vi "Low-Level Write.vi"(5 "Finished? (True)":bool=TRUE, 6 "Mask payload?":bool, 7 "Opcode (Text)":T1=1 items=["Cont. Frame"=0, "Text"=1, "Binary"=2, "Ping"=9, "Pong"=10], 8 "error in (no error)":errorcluster, 9 "timeout ms (5000)":i32=5000, 10 "Data":u8[](array[numeric]), 11 "WebSockets in":refnum<class "WebSocket.lvclass">) -> (0 "error out":errorcluster, 1 "timed out?":bool, 3 "WebSockets out":refnum<class "WebSocket.lvclass">)   [LabVIEW 2021, in "WebSockets.lvlib" / "WebSocket.lvclass"]
doc: "Sends a WebSocket frame to the connection endpoint. Messages sent from the client must be masked but it is optional for the server.\n\nFinished should be set to True unless sending a fragmented message.\nWebSockets 2.0.1.40\nSam Sharp - MediaMongrels Ltd\nCopyright (c) 2019, MediaMongrels Ltd"
uses:
  WebSocket.lvclass
  Opcodes.ctl
  WebSocket.lvclass/WebSocket.ctl
  Sockets/Socket/Socket.lvclass
panel:
  # "(leave as 'True' unless sending fragmented messages)"
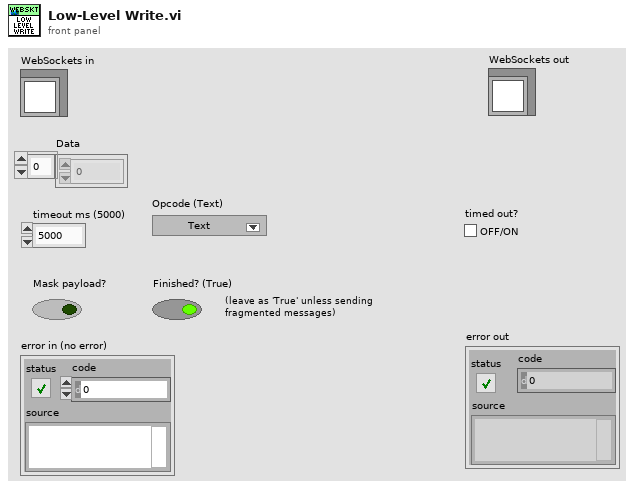
[diagram p1: front panel]
types:
  T1 = typedef "WebSockets.lvlib/WebSocket.lvclass/Opcodes.ctl" = u8
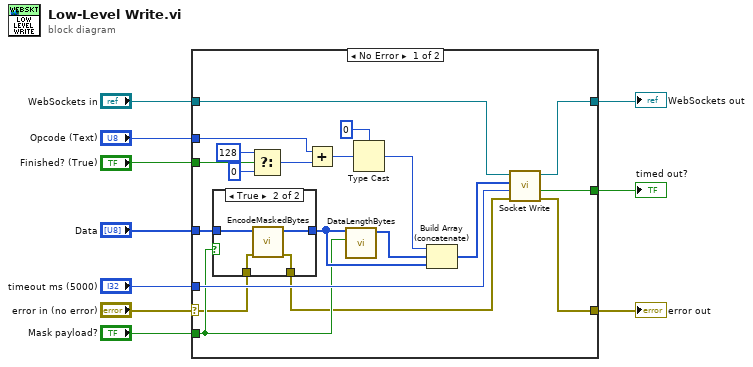
[diagram p0: block diagram]
diagram:
  n1 = case shown="No Error" "error in (no error)" {
    selector: "error in (no error)" -> [w22 w38]
    tunnel: [w30 w38] -> w9
    tunnel: [w12 w37] -> w3
    tunnel: "WebSockets in" -> [w13 w37]
    tunnel: "Data" -> [w25 _]
    tunnel: "timeout ms (5000)" -> [w26 _]
    tunnel: "Mask payload?" -> [w23 _]
    tunnel: "Finished? (True)" -> [w20 _]
    tunnel: "Opcode (Text)" -> [w18 _]
    tunnel: [w11 _] -> w1
    frame No Error {
      n2 = case shown="True" w23 {
        tunnel: w25 -> [w32 w36]
        tunnel: [w32 w35] -> w24
        tunnel: w22 -> [w31 w34]
        tunnel: [w31 w33] -> w21
        frame False {
        }
        frame True {
          n3 = call "EncodeMaskedBytes.vi"("error in (no error)"=w34, "Raw Data"=w36) -> ("error out"=w33:errorcluster, "Masked Data"=w35:u8[])  [unwired: 8 in]
        }
      }
      n4 = Select(t=u8 128, s=w20, f=u8 0) -> (s? t:f=w19:u8)
      n5 = Add(x=w18, y=w19) -> (x+y=w28:T1)
      n6 = call "DataLengthBytes.vi"("Is masked?"=w23, "Data"=w24) -> ("Length Bytes"=w29:u8[])  [unwired: 9 in]
      n7 = Type Cast(type=u8 0 ("f"), x=w28) -> (*(type *) &x=w15:u8)
      n8 = Build Array (concatenate)(w15, w29, w24) -> (w27:u8[])
      n9 = call "Socket Write.vi"("error in (no error)"=w21, "timeout ms (5000)"=w26, "Bytes to write"=w27, "WebSocket in"=w13) -> ("error out"=w30:errorcluster, "timed out?"=w11:bool, "WebSocket out"=w12:refnum<class "WebSocket.lvclass">)  [unwired: 4 in, 1 out]
    }
    frame Error {
    }
  }
  "error out" <- w9
  "WebSockets out" <- w3
  "timed out?" <- w1
